vi "Get Template Path.vi"(11 "Coupled Message Scripter in":refnum<class "Coupled Message Scripter.lvclass">) -> (2 "Template Path":path)   [LabVIEW 2020, in "Message Maker.lvlib" / "Coupled Message Scripter.lvclass"]
uses:
  Coupled Message Scripter.lvclass
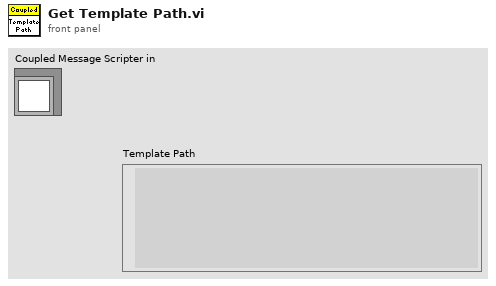
[diagram p1: front panel]
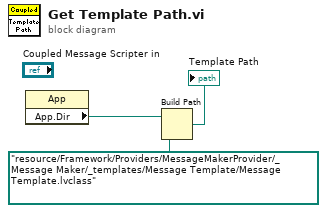
[diagram p0: block diagram]
diagram:
  n1 = property class="App"() -> ("App.Dir"=w1:path)  [unwired: 2 in, 2 out]
  n2 = Build Path(base path=w1, name or relative path=path "resource/Framework/Providers/MessageMakerProvider/_Message Maker/_templates/Message Template/Message Template.lvclass" ("class path")) -> (appended path=→"Template Path":path)
